vi "CALC_MARK_SET.vi"(0 "VISA IN":refnum<visa-resource-name>, 1 "Marker number":i32, 2 "Type":string, 5 "error in":errorcluster, 7 "Channel":i32) -> (14 "VISA Out":refnum<visa-resource-name>, 19 "error out":errorcluster)   [LabVIEW 2018, in "PNA-X.lvlib"]
doc: "CALCulate<cnum>:MARKer<mkr>:SET <char> \n(Write-only) Sets the selected instrument setting to assume the value of the specified marker. \nMarker Functions CENT, SPAN, STARt, and STOP do not work with channels that are in CW or \nSegment Sweep mode. \nSee Critical Note \nParameters \n<cnum> Channel number of the measurement. There must be a selected measurement \non that channel. If unspecified, <cnum> is set to 1. \n<mkr> Any marker number from 1 to 10; if unspecified, value is set to 1 \n<char> Choose from: \nCENTer - changes center frequency to the value of the marker \nSPAN - changes the sweep span to the span that is defined by the delta marker \nand the marker that it references. Unavailable if there is no delta marker. \nSTARt - changes the start frequency to the value of the marker \nSTOP - changes the stop frequency to the value of the marker \nRLEVel - changes the reference level to the value of the marker \nDELay - changes the line length at the receiver input to the phase slope at the \nactive marker stimulus position. \nExamples CALC:MARK:SET CENT \ncalculate2:marker8:set span \nQuery Syntax Not Applicable \nDefault Not Applicable"
uses:
  PNA-X.lvlib
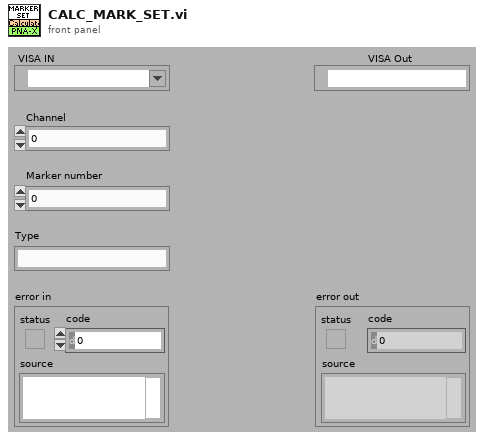
[diagram p1: front panel]
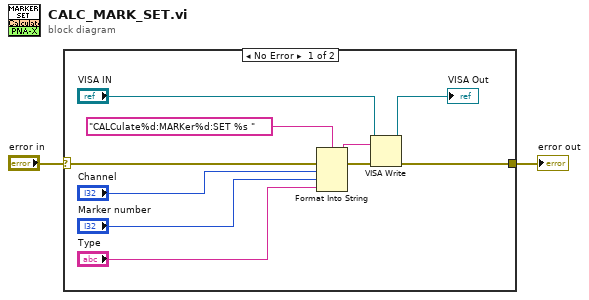
[diagram p0: block diagram]
diagram:
  n1 = case shown="No Error" "error in" {
    selector: "error in" -> [w12 w13]
    tunnel: [w7 w13] -> w1
    frame No Error {
      n2 = Format Into String(format string="CALCulate%d:MARKer%d:SET %s " ("Cmdline"), error in=w12, "Channel", "Marker number", "Type") -> (resulting string=w10:string, error out=w11:errorcluster)  [unwired: 1 in]
      n3 = VISA Write(VISA resource name="VISA IN", write buffer=w10, error in (no error)=w11) -> (VISA resource name out=→"VISA Out":refnum<visa-resource-name>, error out=w7:errorcluster)  [unwired: 1 out]
    }
    frame Error {
    }
  }
  "error out" <- w1
